vi "PIV_Stats_Single.vi"(0 "Data Folder":path=path "T:/Ensight_Data/NACA0015/NACA0015_NM_B/Test_A", 1 "PIV Meas Plane":enum16{"XY", "YZ", "XZ"}(ring)=enum."XZ", 2 "Row number":i32=1, 5 "Output Directory":path=path "T:/Ensight_Data/NACA0015/NACA0015_NM_B", 7 "XYZ Translation":dbl[](array[numeric])=[200.0, 8.0, -30.0], 9 "Case Name":string="Test_A_Case", 11 "PIV Freq (Hz)":dbl=7.25, 12 "Invert U":bool=TRUE, 13 "Invert V":bool) -> (4 "Progress Bar":i32(slide) scale=0.0..100.0, 6 "Status":string, 10 "# total vectors":i32=9858)   [LabVIEW 2011]
uses:
  <vilib>/Utility/error.llb/DialogType.ctl
  <vilib>/Analysis/1siggen.llb/Ramp Pattern by Samples.vi
  <vilib>/Analysis/NI_AALBase.lvlib
panel:
  out "Max Record Length":i32=3
  out "Tmax":dbl=0.41379310344827586
  out "# vectors without records":i16
  out "Data Array (spot,Var)":dbl[][](array[numeric])
  out "File Paths":path[](array[path])
  out "Position Array (XYZ,spot)":dbl[][](array[numeric])
  out "Variable Names":string[](array[string])=["Record_Length", "CHC", "u_ms", "v_ms", "time_s", "Vel_mag_ms", "Turb_Stats_U_ms", "Turb_Stats_u2_m2s2", "Turb_Stats_u3_m3s3", "Turb_Stats_u4_m4s4", "Turb_Stats_TurbU_%", "Turb_Stats_Skew_u", "Turb_Stats_Kurt_u", "Turb_Stats_V_ms", "Turb_Stats_v2_m2s2", "Turb_Stats_v3_m3s3", "Turb_Stats_v4_m4s4", "Turb_Stats_TurbV_%", "Turb_Stats_Skew_v", "Turb_Stats_Kurt_v", "Turb_Stats_u2v2_m4s4", "Turb_Stats_uv3_m4s4", "Turb_Stats_u3v_m4s4", "Turb_Stats_uv2_m3s3", "Turb_Stats_u2v_m3s3", "Turb_Stats_uv_cc", "Turb_Stats_uv", "Turb_Stats_TKE_J", "Turb_Stats_Error_U_ms", "Turb_Stats_Error_u2_m2s2", "Turb_Stats_Error_u3_m3s3", "Turb_Stats_Error_u4_m4s4", "Turb_Stats_Error_TurbU_%", "Turb_Stats_Error_Skew_u", "Turb_Stats_Error_Kurt_u", "Turb_Stats_Error_V_ms", "Turb_Stats_Error_v2_m2s2", "Turb_Stats_Error_v3_m3s3", "Turb_Stats_Error_v4_m4s4", "Turb_Stats_Error_TurbV_%", "Turb_Stats_Error_Skew_v", "Turb_Stats_Error_Kurt_v", "Turb_Stats_Error_u2v2_m4s4", "Turb_Stats_Error_uv3_m4s4", "Turb_Stats_Error_u3v_m4s4", "Turb_Stats_Error_uv2_m3s3", "Turb_Stats_Error_u2v_m3s3", "Turb_Stats_Error_uv_cc", "Turb_Stats_Error_uv", "Turb_Stats_Error_TKE_J"]
  out "time s":dbl[](array[numeric])=[0.0, 0.20689655172413793, 0.41379310344827586]
  out "File Array":path[](array[path])=[path "T:/Ensight_Data/NACA0015/NACA0015_NM_A/Test_A_Trans/New folder/Test_A000000.T076.D000.P000.H000.L.vec", path "T:/Ensight_Data/NACA0015/NACA0015_NM_A/Test_A_Trans/New folder/Test_A000001.T076.D000.P000.H000.L.vec", path "T:/Ensight_Data/NACA0015/NACA0015_NM_A/Test_A_Trans/New folder/Test_A000002.T076.D000.P000.H000.L.vec"]
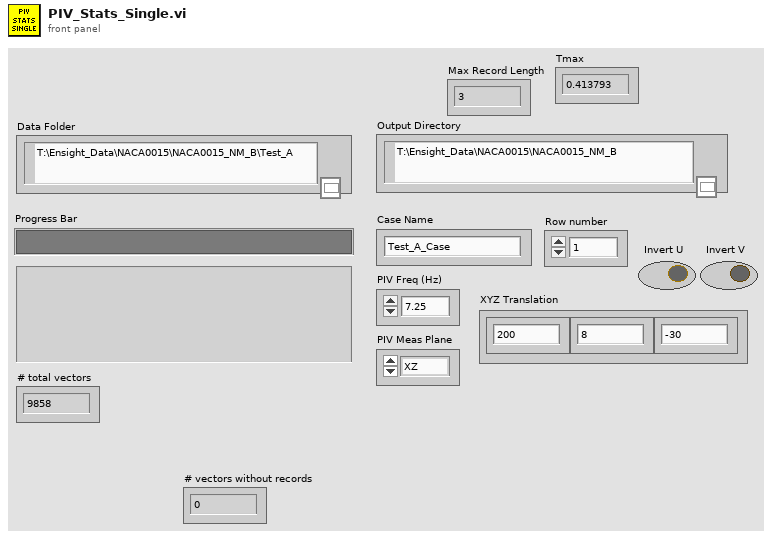
[diagram p1: front panel]
types:
  T1 = cluster{"Record Length":dbl, "CHC":dbl[], "u m/s":dbl[], "v m/s":dbl[], "time s":dbl[], "Vel mag m/s":dbl[], "XYZ Position":dbl[], " Turb Stats":cluster{"U m/s":dbl, "u2 m2/s2":dbl, "u3 m3/s3":dbl, "u4 m4/s4":dbl, "TurbU %":dbl, "Skew_u":dbl, "Kurt_u":dbl, "V m/s":dbl, "v2 m2/s2":dbl, "v3 m3/s3":dbl, "v4 m4/s4":dbl, "TurbV %":dbl, "Skew_v":dbl, "Kurt_v":dbl, "u2v2 m4/s4":dbl, "uv3 m4/s4":dbl, "u3v m4/s4":dbl, "uv2 m3/s3":dbl, "u2v m3/s3":dbl, "uv_cc":dbl, "uv":dbl, "TKE J":dbl}[], "Turb Stats Error":cluster{"U m/s":dbl, "u2 m2/s2":dbl, "u3 m3/s3":dbl, "u4 m4/s4":dbl, "TurbU %":dbl, "Skew_u":dbl, "Kurt_u":dbl, "V m/s":dbl, "v2 m2/s2":dbl, "v3 m3/s3":dbl, "v4 m4/s4":dbl, "TurbV %":dbl, "Skew_v":dbl, "Kurt_v":dbl, "u2v2 m4/s4":dbl, "uv3 m4/s4":dbl, "u3v m4/s4":dbl, "uv2 m3/s3":dbl, "u2v m3/s3":dbl, "uv_cc":dbl, "uv":dbl, "TKE J":dbl}[], "u (good)":dbl[], "v (good)":dbl[]}
  T2 = cluster{"Record Length":dbl, "CHC":dbl[], "u m/s":dbl[], "v m/s":dbl[], "time s":dbl[], "Vel mag m/s":dbl[], "XYZ Position":dbl[], " Turb Stats":cluster{"U m/s":dbl, "u2 m2/s2":dbl, "u3 m3/s3":dbl, "u4 m4/s4":dbl, "TurbU %":dbl, "Skew_u":dbl, "Kurt_u":dbl, "V m/s":dbl, "v2 m2/s2":dbl, "v3 m3/s3":dbl, "v4 m4/s4":dbl, "TurbV %":dbl, "Skew_v":dbl, "Kurt_v":dbl, "u2v2 m4/s4":dbl, "uv3 m4/s4":dbl, "u3v m4/s4":dbl, "uv2 m3/s3":dbl, "u2v m3/s3":dbl, "uv_cc":dbl, "uv":dbl, "TKE J":dbl}[], "Turb Stats Error":cluster{"U m/s":dbl, "u2 m2/s2":dbl, "u3 m3/s3":dbl, "u4 m4/s4":dbl, "TurbU %":dbl, "Skew_u":dbl, "Kurt_u":dbl, "V m/s":dbl, "v2 m2/s2":dbl, "v3 m3/s3":dbl, "v4 m4/s4":dbl, "TurbV %":dbl, "Skew_v":dbl, "Kurt_v":dbl, "u2v2 m4/s4":dbl, "uv3 m4/s4":dbl, "u3v m4/s4":dbl, "uv2 m3/s3":dbl, "u2v m3/s3":dbl, "uv_cc":dbl, "uv":dbl, "TKE J":dbl}[], "u (good)":dbl[], "v (good)":dbl[]}[]
  T3 = cluster{"U m/s":dbl, "u2 m2/s2":dbl, "u3 m3/s3":dbl, "u4 m4/s4":dbl, "TurbU %":dbl, "Skew_u":dbl, "Kurt_u":dbl, "V m/s":dbl, "v2 m2/s2":dbl, "v3 m3/s3":dbl, "v4 m4/s4":dbl, "TurbV %":dbl, "Skew_v":dbl, "Kurt_v":dbl, "u2v2 m4/s4":dbl, "uv3 m4/s4":dbl, "u3v m4/s4":dbl, "uv2 m3/s3":dbl, "u2v m3/s3":dbl, "uv_cc":dbl, "uv":dbl, "TKE J":dbl}
  T4 = cluster{"U m/s":dbl, "u2 m2/s2":dbl, "u3 m3/s3":dbl, "u4 m4/s4":dbl, "TurbU %":dbl, "Skew_u":dbl, "Kurt_u":dbl, "V m/s":dbl, "v2 m2/s2":dbl, "v3 m3/s3":dbl, "v4 m4/s4":dbl, "TurbV %":dbl, "Skew_v":dbl, "Kurt_v":dbl, "u2v2 m4/s4":dbl, "uv3 m4/s4":dbl, "u3v m4/s4":dbl, "uv2 m3/s3":dbl, "u2v m3/s3":dbl, "uv_cc":dbl, "uv":dbl, "TKE J":dbl}[]
  T5 = typedef "DialogType.ctl" = u16
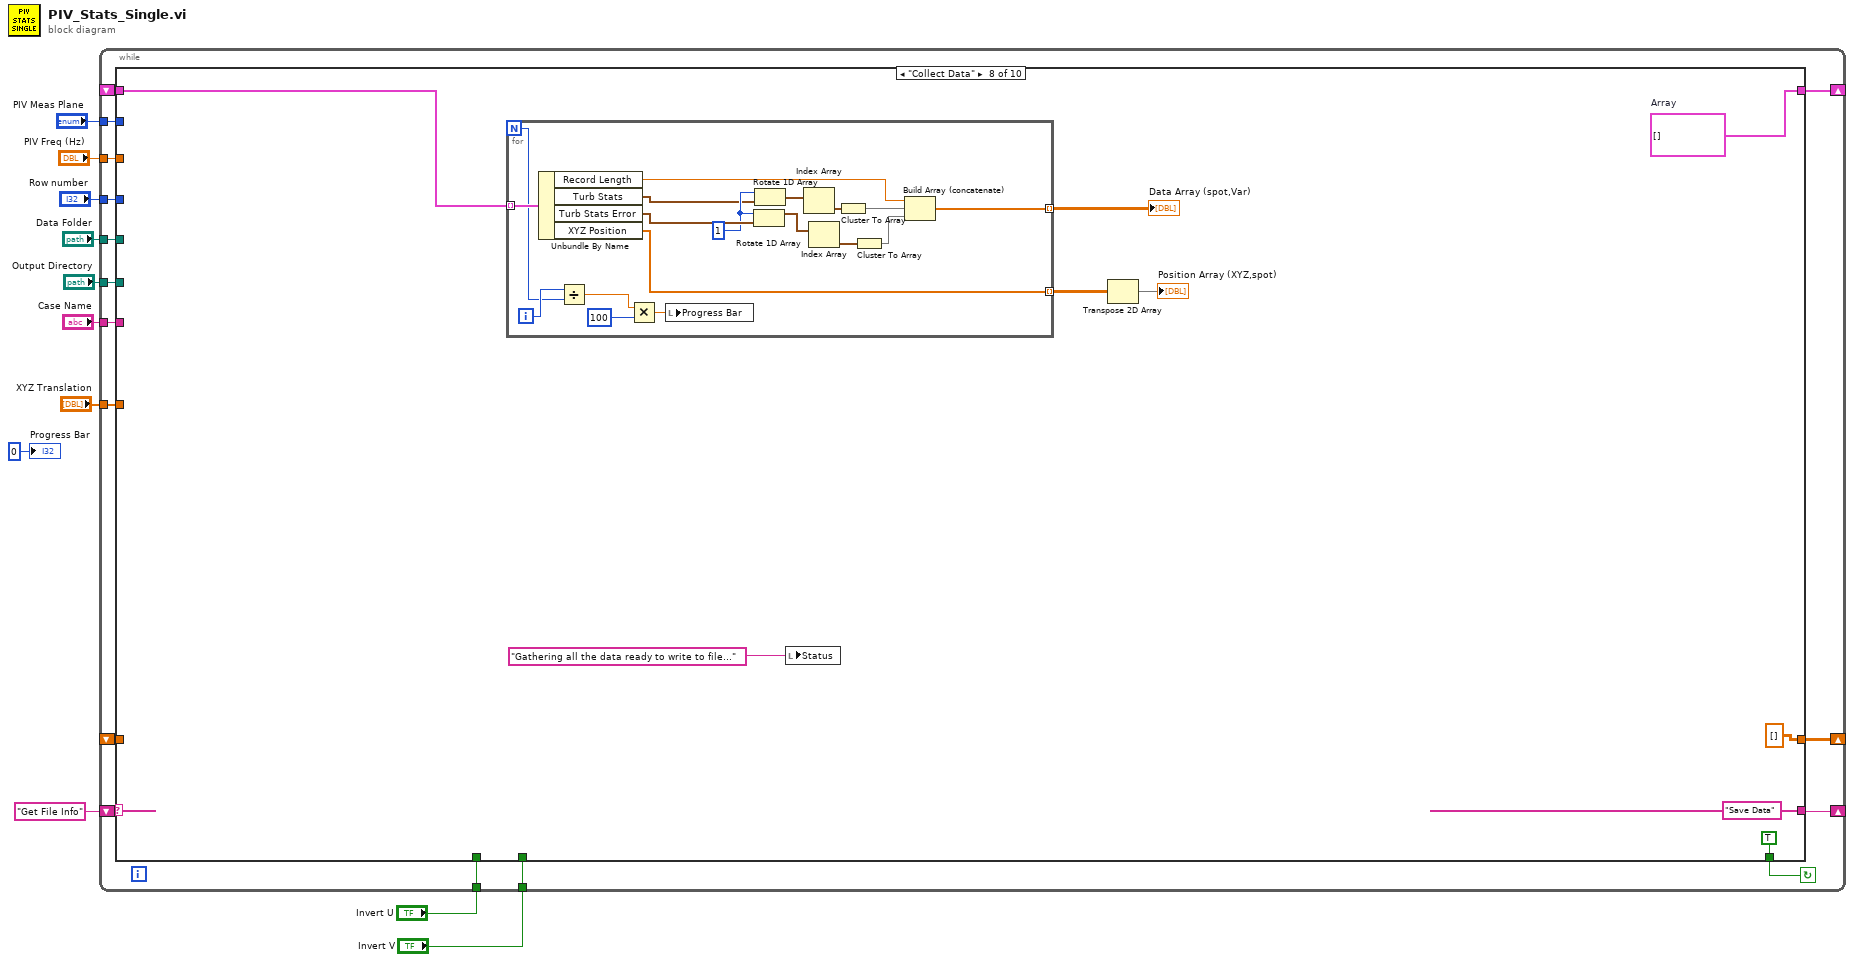
[diagram p0: block diagram]
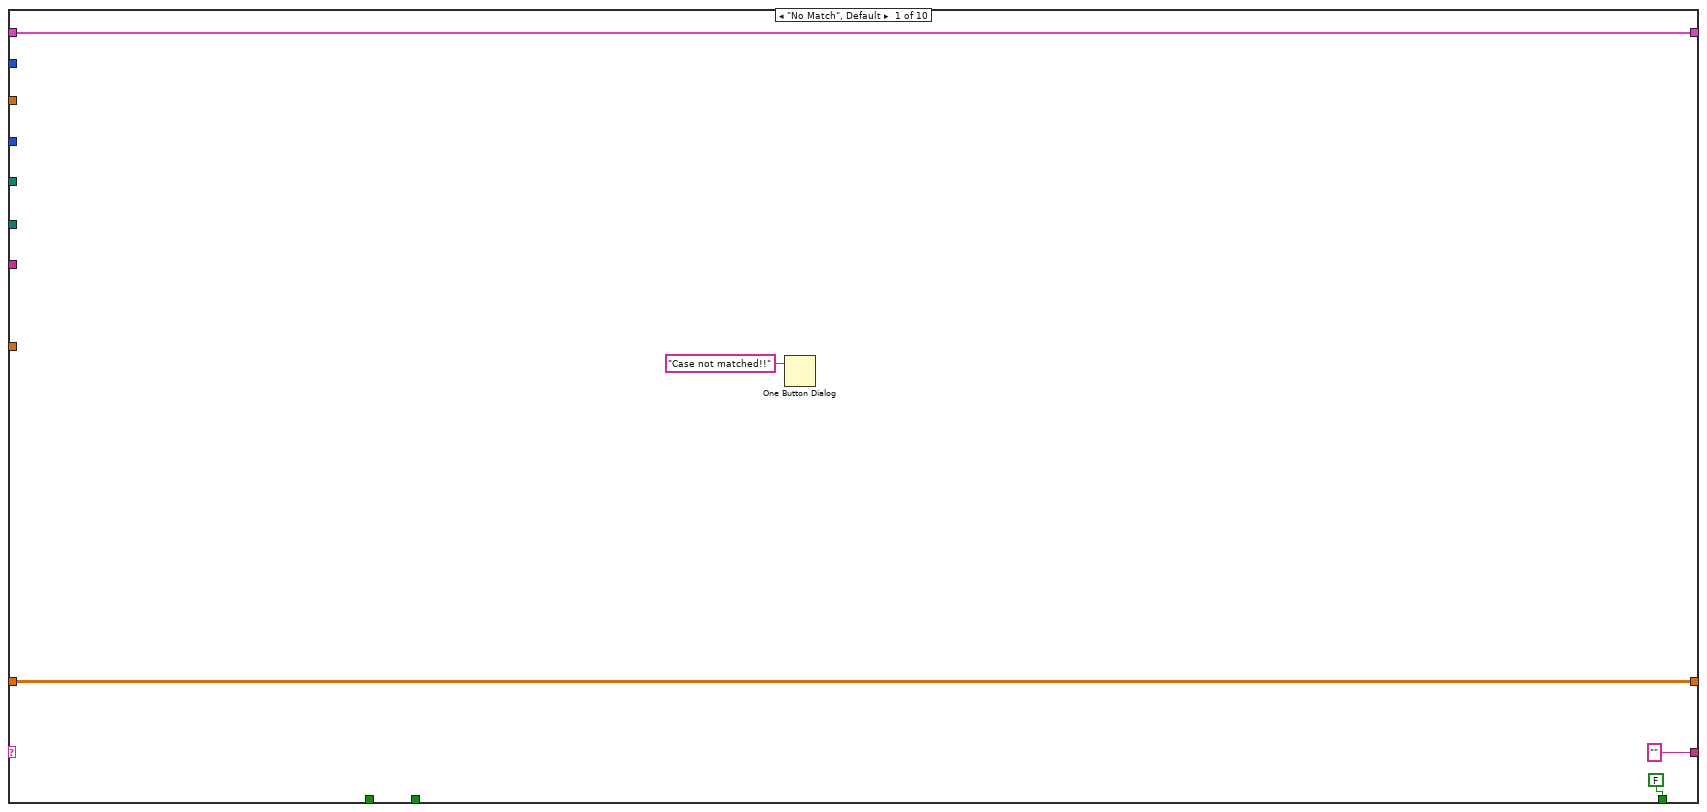
[diagram p2: hidden frame]
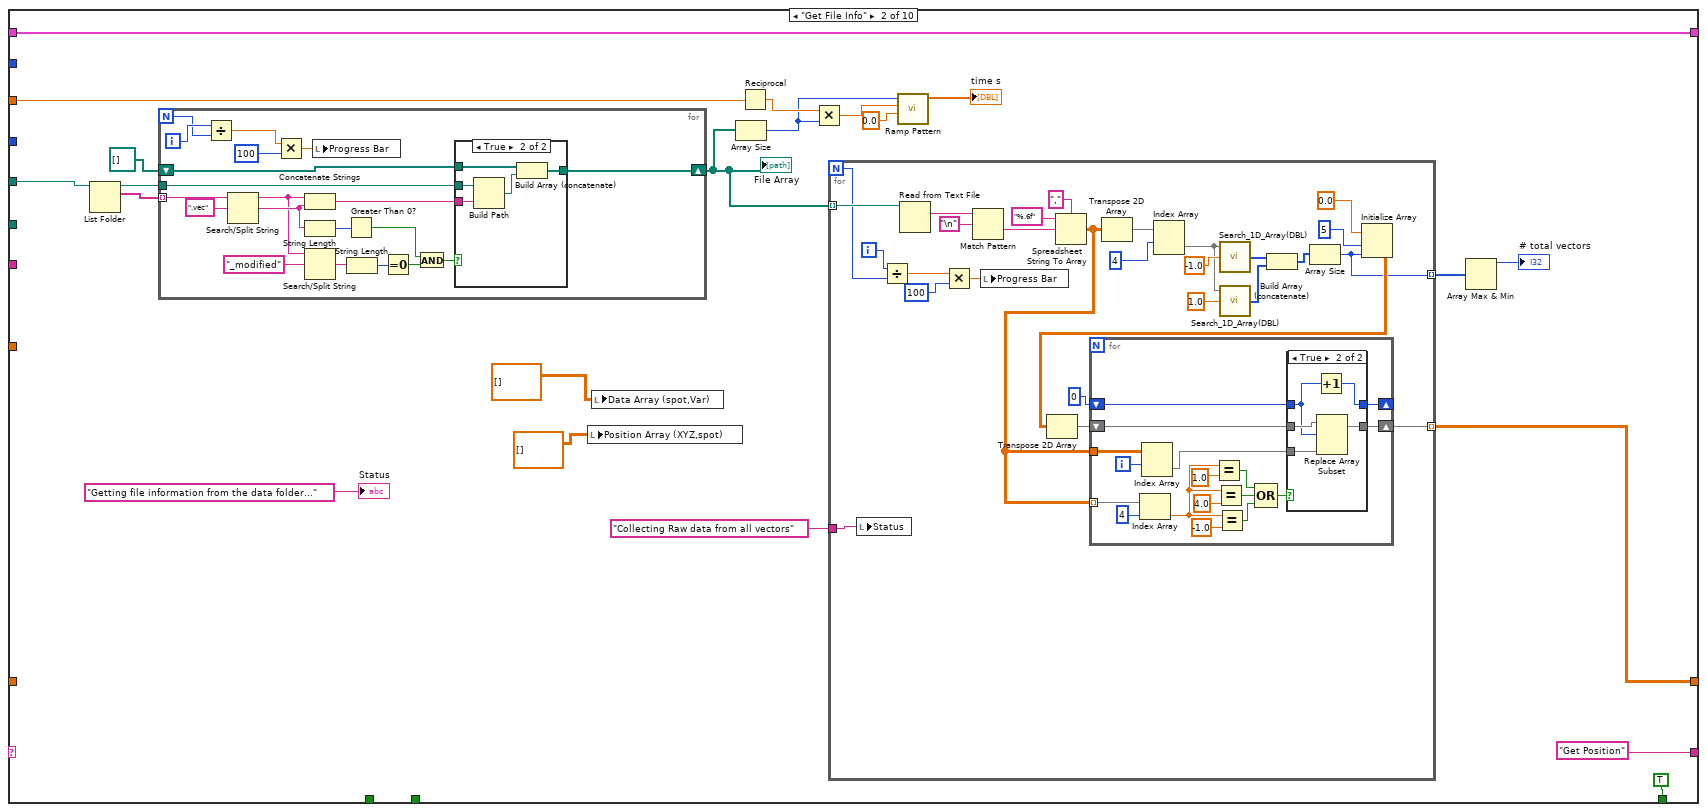
[diagram p3: hidden frame]
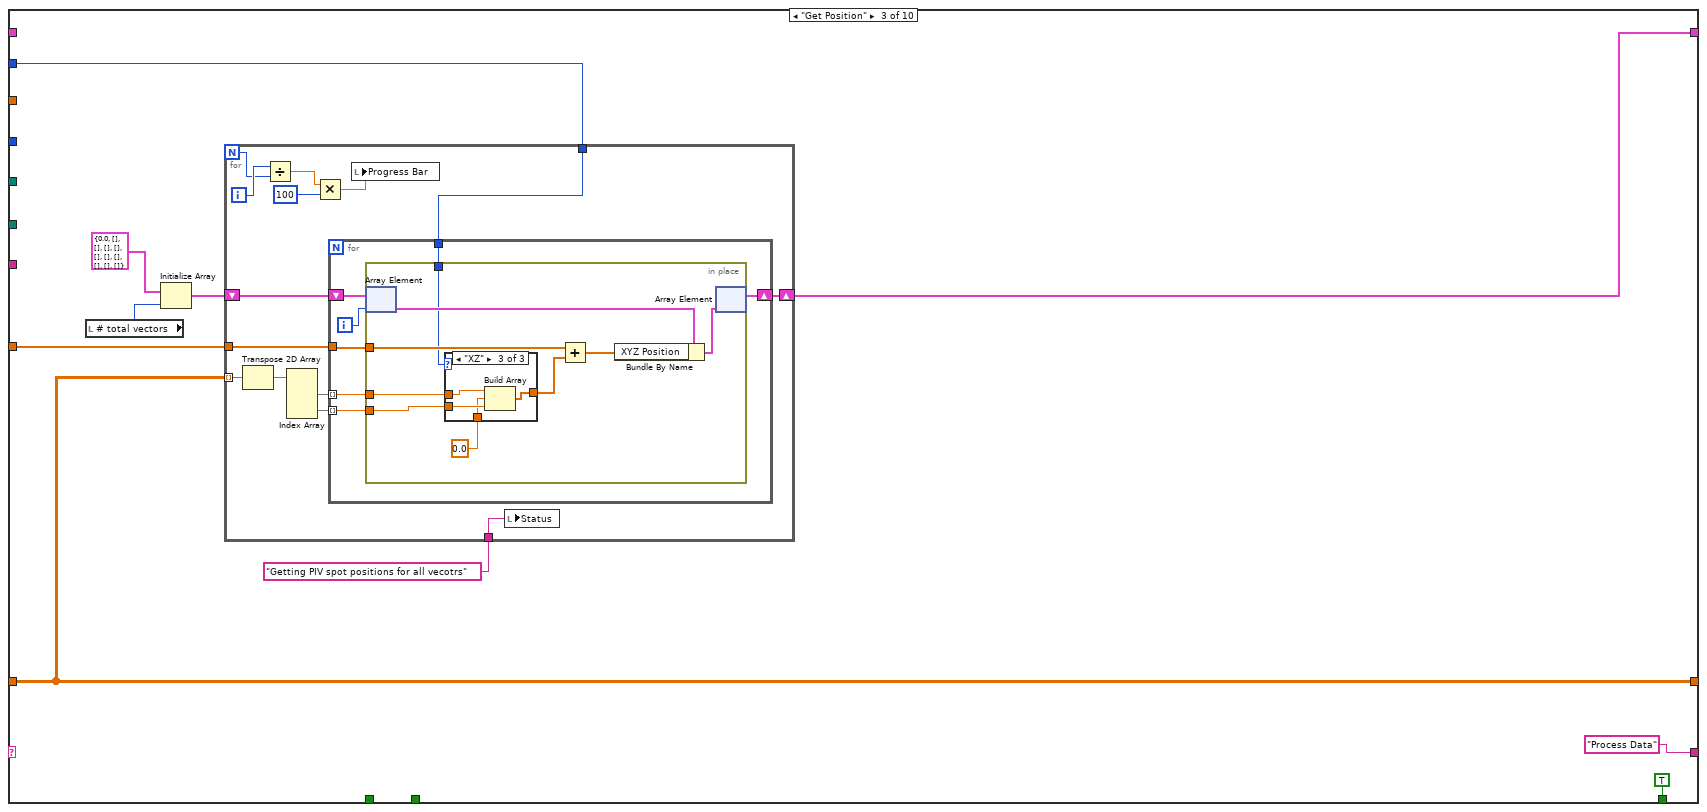
[diagram p6: hidden frame]
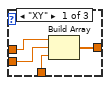
[diagram p7: hidden frame]
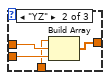
[diagram p8: hidden frame]
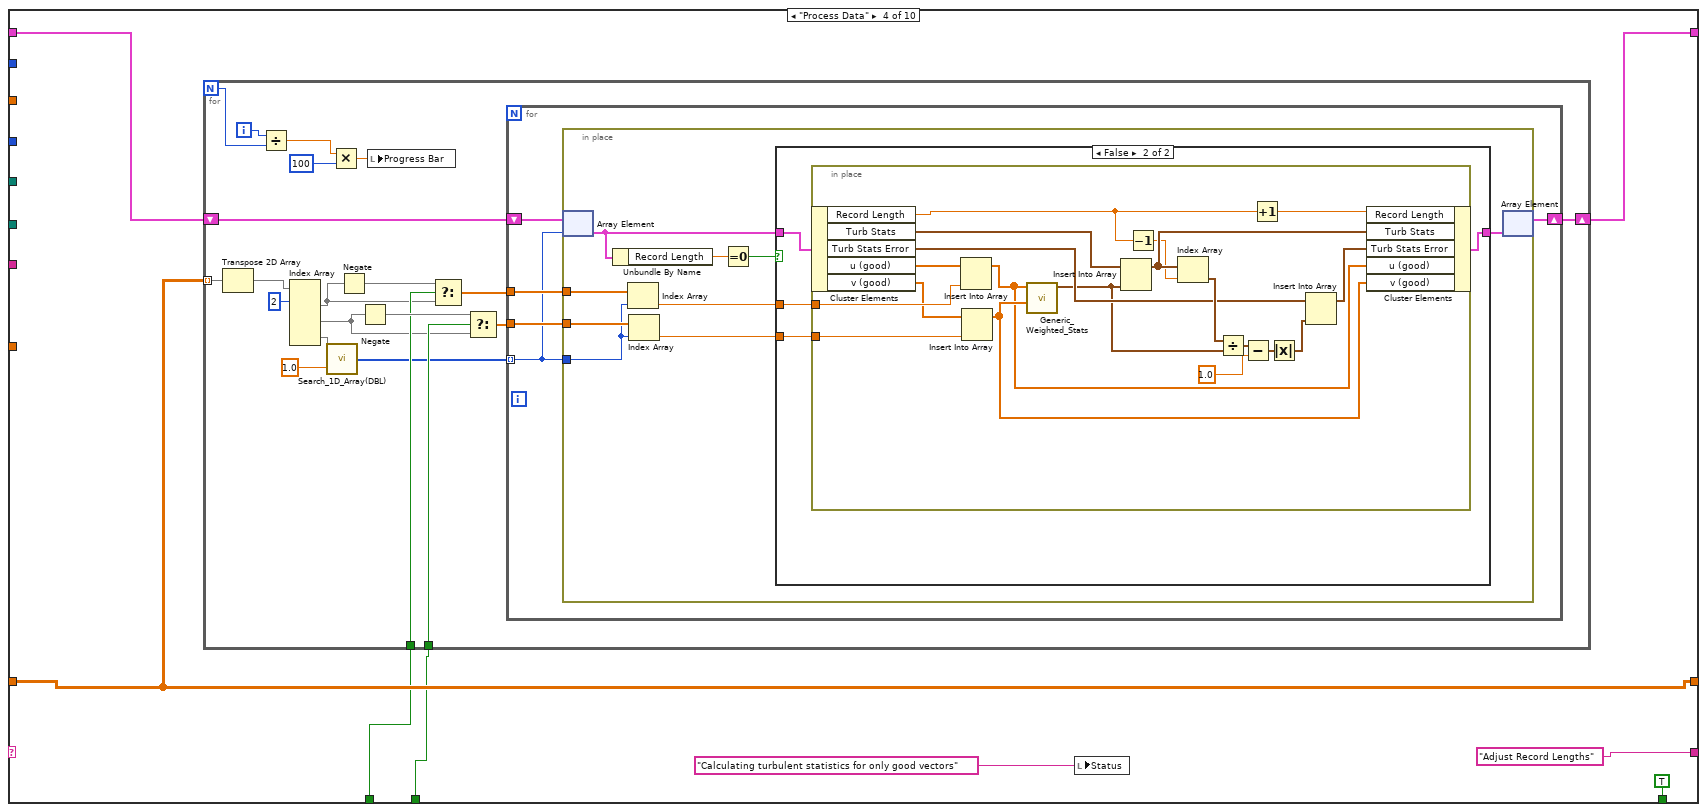
[diagram p9: hidden frame]
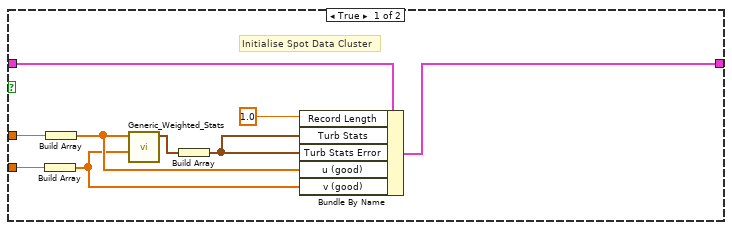
[diagram p10: hidden frame]
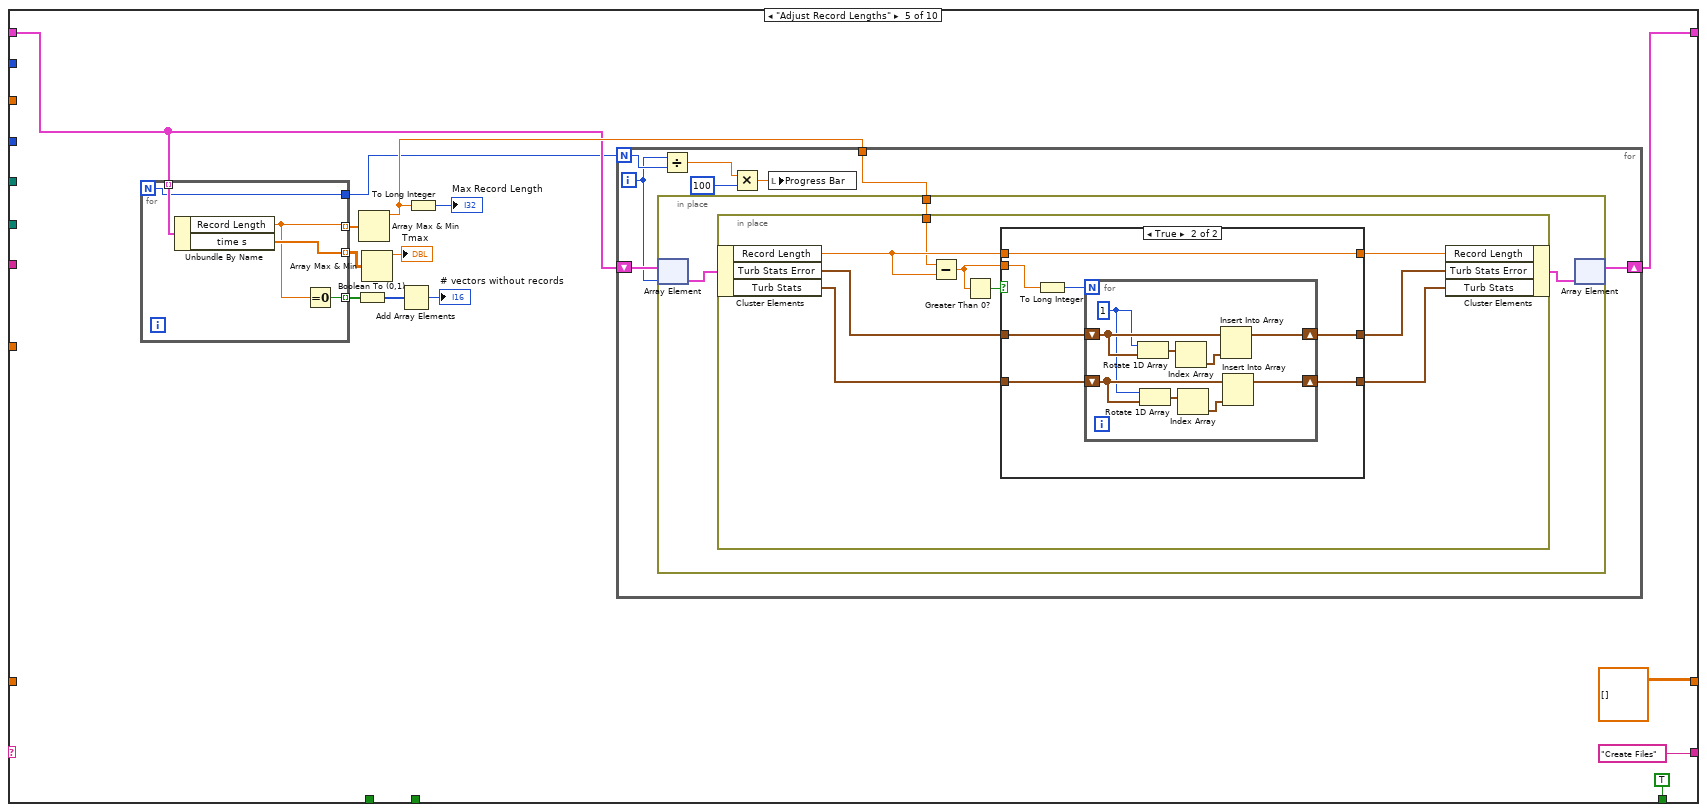
[diagram p11: hidden frame]
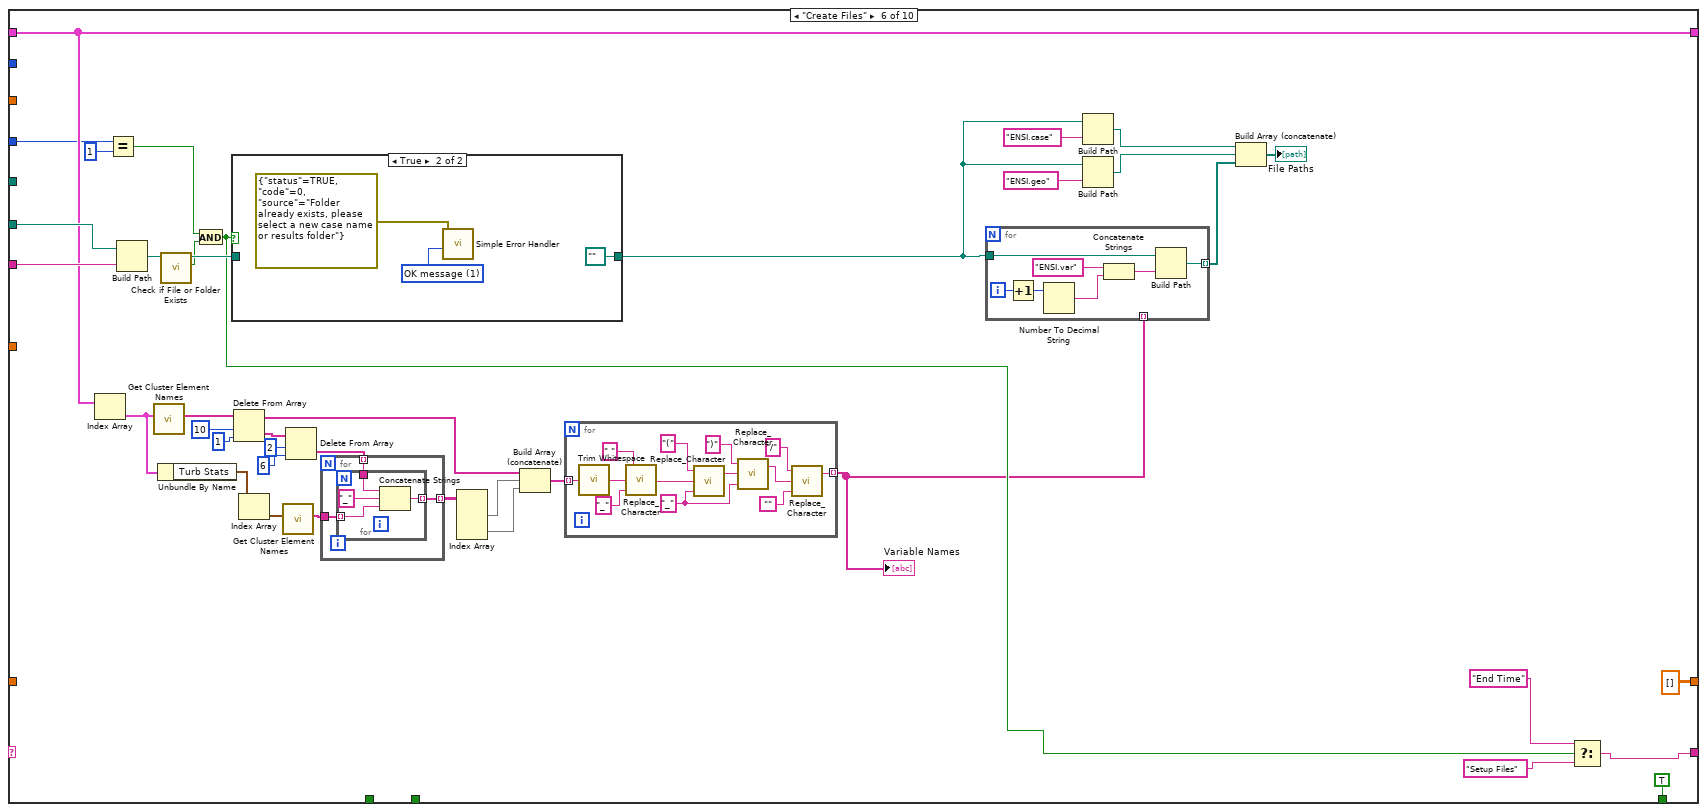
[diagram p13: hidden frame]
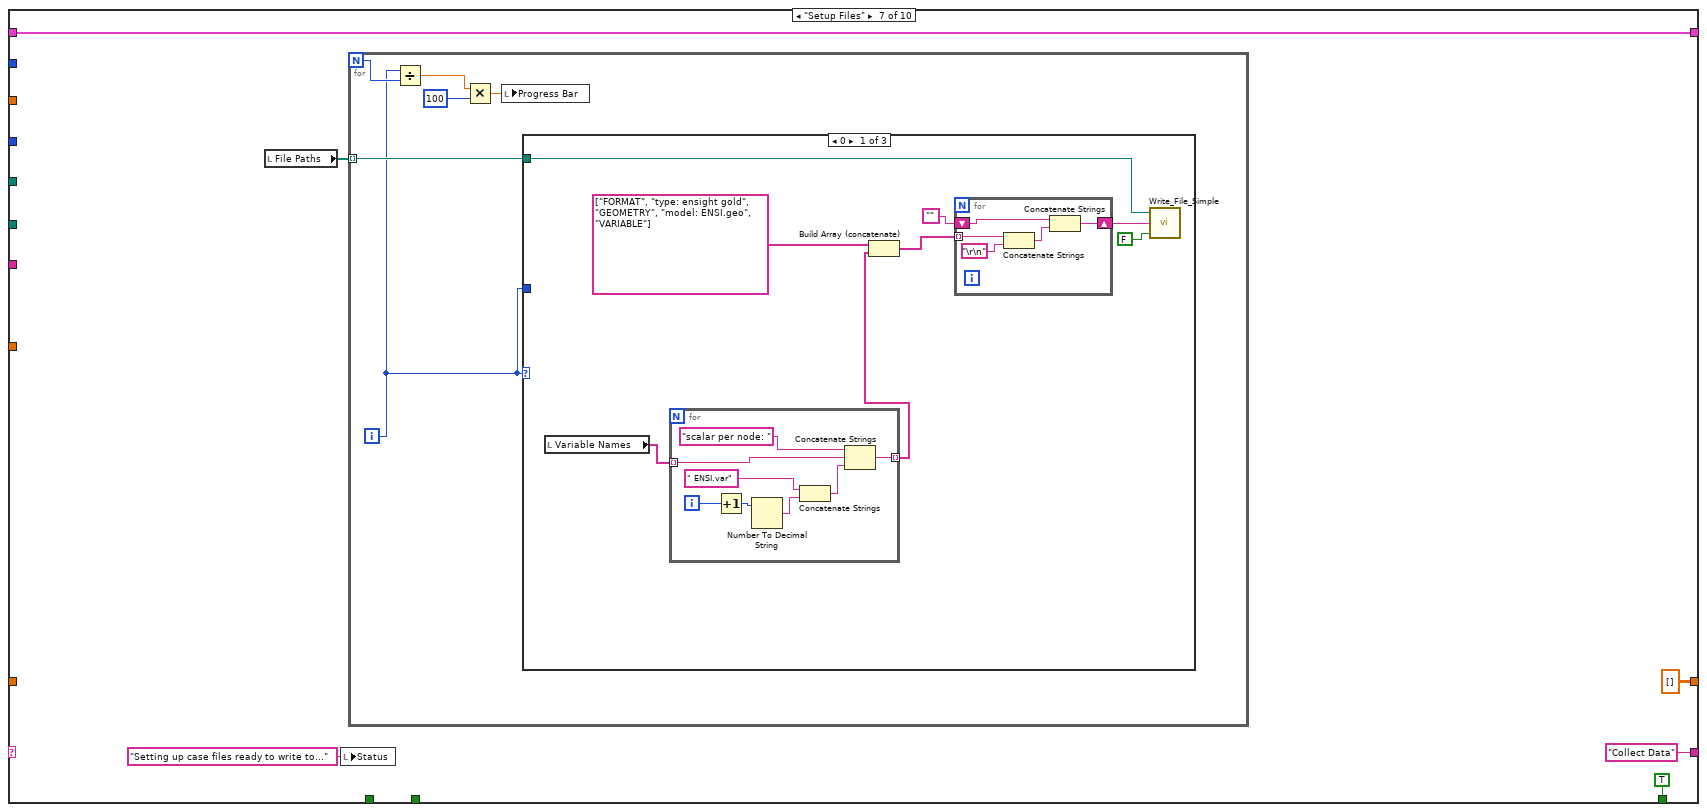
[diagram p15: hidden frame]
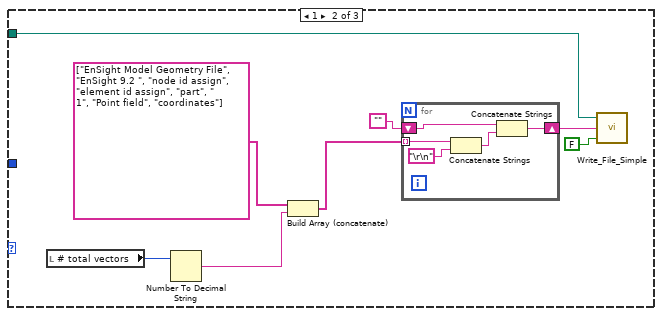
[diagram p16: hidden frame]
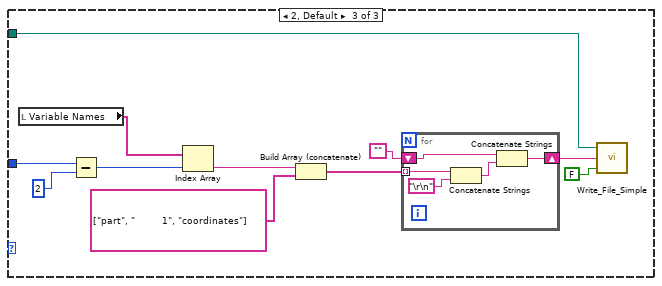
[diagram p17: hidden frame]
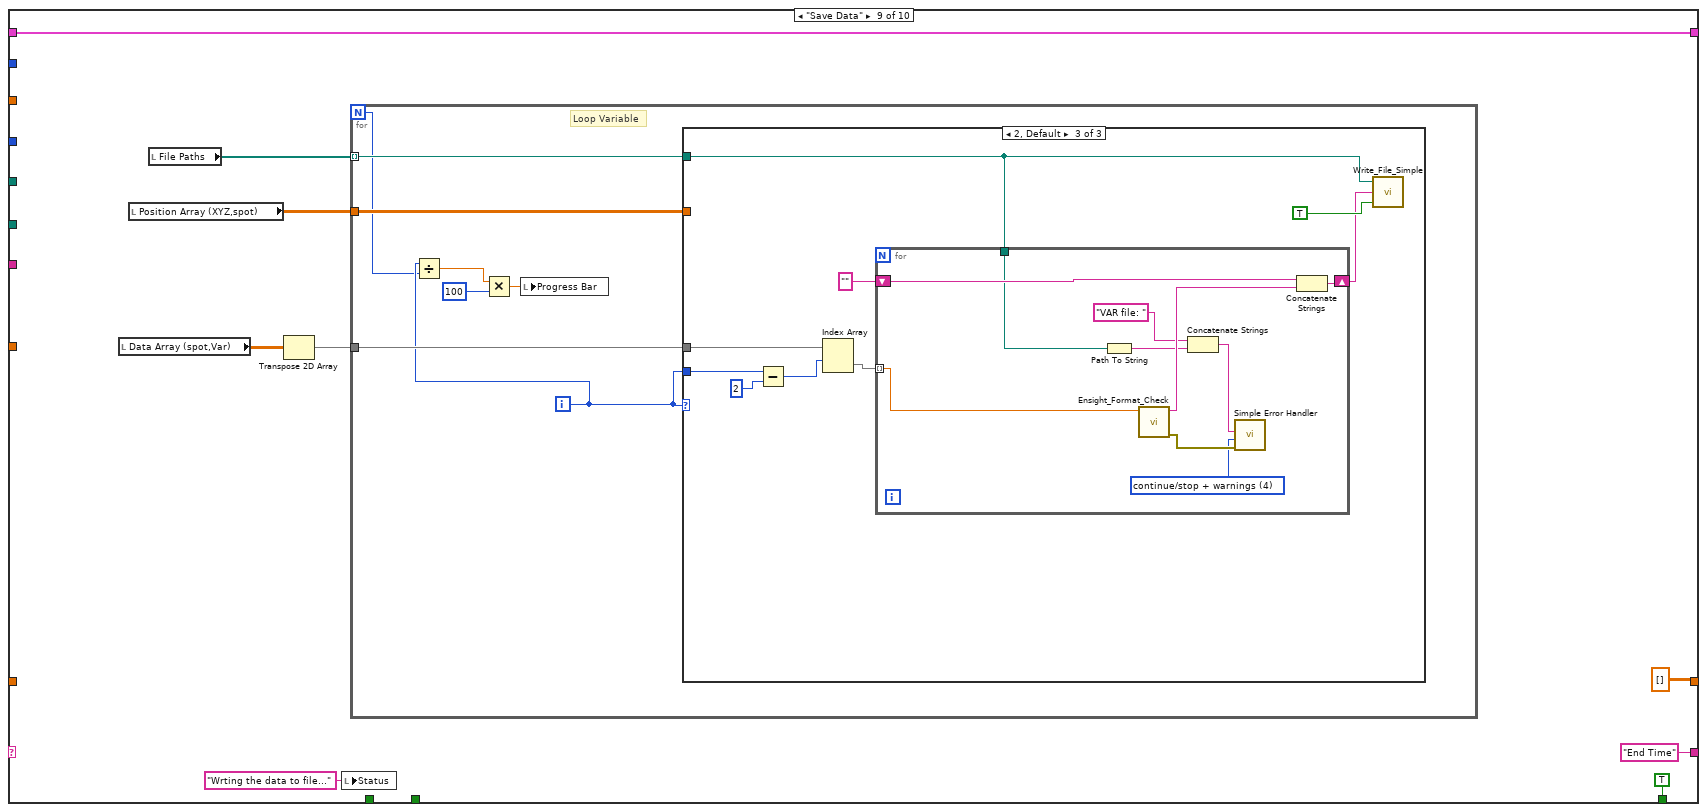
[diagram p18: hidden frame]
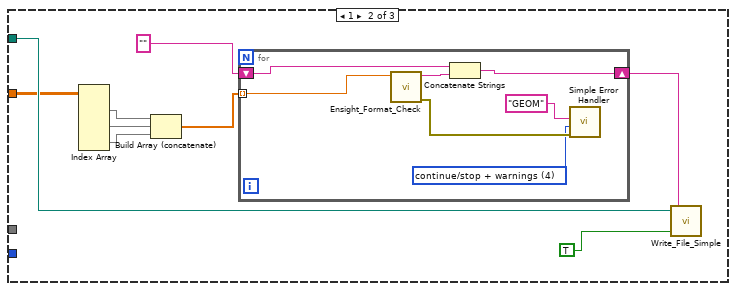
[diagram p20: hidden frame]
diagram:
  n1 = while {
    shift-right: [w26] -> _
    shift-left: "Get File Info" -> [w27]
    tunnel: "Data Folder" -> [w25]
    tunnel: "Output Directory" -> [w23]
    tunnel: "Case Name" -> [w22]
    tunnel: "PIV Freq (Hz)" -> [w21]
    tunnel: "PIV Meas Plane" -> [w20]
    tunnel: "XYZ Translation" -> [w19]
    shift-right: [w18] -> _
    shift-left: _ -> [w17]
    tunnel: "Row number" -> [w16]
    tunnel: "Invert V" -> [w15]
    tunnel: "Invert U" -> [w14]
    shift-right: [w13] -> _
    shift-left: _ -> [w12]
    stop <- w24 continue-if-true
    n2 = case shown="\"Collect Data\"" w27 {
      tunnel: ["" "Get Position" "Process Data" "Adjust Record Lengths" "Create Files" w330 "Collect Data" ("t") "Save Data" ("t") "End Time" ("t") "" ("t")] -> w26
      tunnel: w25 -> [_ w48 _ _ _ _ _ _ _ _]
      tunnel: [FALSE TRUE TRUE TRUE TRUE TRUE TRUE TRUE TRUE FALSE] -> w24
      tunnel: w23 -> [_ _ _ _ _ w354 _ _ _ _]
      tunnel: w22 -> [_ _ _ _ _ w355 _ _ _ _]
      tunnel: w21 -> [_ w47 _ _ _ _ _ _ _ _]
      tunnel: w20 -> [_ _ w138 _ _ _ _ _ _ _]
      tunnel: w19 -> [_ _ w139 _ _ _ _ _ _ _]
      tunnel: [w30 w35 w133 w184 w260 w340 w389 w453 w482 w529] -> w18
      tunnel: w17 -> [w30 w35 _ w188 w262 w340 w389 w455 w482 w529]
      tunnel: w16 -> [_ _ _ _ _ w336 _ _ _ _]
      tunnel: w15 -> [_ _ _ w185 _ _ _ _ _ _]
      tunnel: w14 -> [_ _ _ w186 _ _ _ _ _ _]
      tunnel: [w28 w33 w132 w187 dbl[][][] [] ("GoodRawData(time,spot)") dbl[][][] [] ("GoodRawData(time,spot)") dbl[][][] [] ("GoodRawData(time,spot)") dbl[][][] [] ("GoodRawData(time,spot)") dbl[][][] [] ("GoodRawData(time,spot)") w528] -> w13
      tunnel: w12 -> [w28 _ w132 w187 _ _ _ _ _ w528]
      frame "No Match", Default {
        n3 = One Button Dialog(message="Case not matched!!") -> ()  [unwired: 1 in, 1 out]
      }
      frame "Get File Info" {
        n4 = List Folder(path=w48) -> (path out=w50:path, filenames=w51:string[])  [unwired: 3 in, 2 out]
        n5 = for {
          N -> [w106]
          tunnel: w51 -> [w125] mode=indexing
          shift-right: [w118] -> w38
          shift-left: path[] [] -> [w120]
          tunnel: w50 -> [w119]
          i -> [w107]
          n6 = Divide(x=w107, y=w106) -> (x/y=w109:dbl)
          n7 = Search/Split String(string=w125, search string/char (-)=".vec") -> (substring before match=w116:string, match + rest of string=w122:string)  [unwired: 1 in, 1 out]
          n8 = Multiply(x=w109, y=100) -> (x*y=w110:dbl)
          n9 = Concatenate Strings(w116, w122) -> (w121:string)
          n10 = String Length(string=w122) -> (length=w123:i32)
          n11 = Search/Split String(string=w116, search string/char (-)="_modified") -> (match + rest of string=w114:string)  [unwired: 1 in, 2 out]
          n12 = local write "Progress Bar"(w110) -> ()
          n13 = Greater Than 0?(x=w123) -> (x > 0?=w117:bool)
          n14 = String Length(string=w114) -> (length=w113:i32)
          n15 = Equal To 0?(x=w113) -> (x = 0?=w112:bool)
          n16 = And(x=w117, y=w112) -> (x .and. y?=w111:bool)
          n17 = case shown="True" w111 {
            tunnel: w121 -> [_ w131]
            tunnel: w120 -> [w126 w127]
            tunnel: w119 -> [_ w130]
            tunnel: [w126 w128] -> w118
            frame False {
            }
            frame True {
              n18 = Build Path(base path=w130, name or relative path=w131) -> (appended path=w129:path)
              n19 = Build Array (concatenate)(w127, w129) -> (w128:path[])
            }
          }
        }
        "File Array" <- w38
        n20 = local write "Position Array (XYZ,spot)"(dbl[][] [] ("Position Array")) -> ()
        n21 = local write "Data Array (spot,Var)"(dbl[][] [] ("Data Array")) -> ()
        n22 = Array Size(array=w38) -> (size(s)=w42:i32)
        n23 = Reciprocal(x=w47) -> (1/x=w45:dbl)
        n24 = Multiply(x=w45, y=w42) -> (x*y=w46:dbl)
        n25 = for {
          N -> [w65]
          tunnel: w38 -> [w72] mode=indexing
          tunnel: [w54] -> w37 mode=indexing
          tunnel: [w69] -> w33 mode=indexing
          tunnel: "Collecting Raw data from all vectors" ("Status") -> [w63]
          i -> [w64]
          n26 = local write "Status"(w63) -> ()
          n27 = Divide(x=w64, y=w65) -> (x/y=w67:dbl)
          n28 = Read from Text File(file (use dialog)=w72) -> (text=w81:string)  [unwired: 3 in, 3 out]
          n29 = Multiply(x=w67, y=100) -> (x*y=w66:dbl)
          n30 = Match Pattern(string=w81, regular expression="\n") -> (after substring=w77:string)  [unwired: 1 in, 3 out]
          n31 = local write "Progress Bar"(w66) -> ()
          n32 = Spreadsheet String To Array(delimiter (Tab)=",", format string="%.6f", spreadsheet string=w77) -> (array=w60:dbl[][])  [unwired: 1 in]
          n33 = Transpose 2D Array(2D array=w60) -> (transposed array=w76:dbl[][])
          n34 = Index Array(array=w76, index (row)=4) -> (element=w59:dbl[])  [unwired: 1 in]
          n35 = call "Search_1D_Array(DBL).vi"("Array"=w59, "Element Data"=-1.0) -> ("Indicies of Elements"=w58:i32[])  [unwired: 7 in]
          n36 = call "Search_1D_Array(DBL).vi"("Array"=w59, "Element Data"=1.0) -> ("Indicies of Elements"=w56:i32[])  [unwired: 7 in]
          n37 = Build Array (concatenate)(w58, w56) -> (w57:i32[])
          n38 = Array Size(array=w57) -> (size(s)=w54:i32)
          n39 = Initialize Array(0.0 ("element"), 5 ("dimension size"), w54) -> (w70:dbl[][])
          n40 = Transpose 2D Array(2D array=w70) -> (transposed array=w71:dbl[][])
          n41 = for {
            tunnel: w60 -> [w93] mode=indexing
            shift-right: [w96] -> w69
            shift-left: w71 -> [w91]
            shift-right: [w95] -> _
            shift-left: 0 ("y") -> [w94]
            tunnel: w60 -> [w92]
            i -> [w90]
            n42 = Index Array(array=w93, index=4) -> (element=w87:dbl)
            n43 = Index Array(array=w92, index (row)=w90) -> (element=w97:dbl[])  [unwired: 1 in]
            n44 = Equal?(x=w87, y=1.0) -> (x = y?=w83:bool)
            n45 = Equal?(x=w87, y=4.0) -> (x = y?=w84:bool)
            n46 = Equal?(x=w87, y=-1.0) -> (x = y?=w85:bool)
            n47 = Compound Arithmetic op=OR(w83, w84, w85) -> (w82:bool)
            n48 = case shown="True" w82 {
              tunnel: w97 -> [_ w103]
              tunnel: w91 -> [w100 w105]
              tunnel: [w100 w104] -> w96
              tunnel: [w99 w102] -> w95
              tunnel: w94 -> [w99 w101]
              frame False {
              }
              frame True {
                n49 = Increment(x=w101) -> (x+1=w102:i32)
                n50 = Replace Array Subset(array=w105, new element=w103, index (row)=w101) -> (w104:dbl[][])  [unwired: 1 in]
              }
            }
          }
        }
        n51 = call-poly <vilib>:"Ramp Pattern.vi"("start"=0.0, "end"=w46, "samples"=w42) -> ("Ramp Pattern"=→"time s":dbl[])  [unwired: 7 in, 1 out]
        n52 = Array Max & Min(array=w37) -> (max value=→"# total vectors":i32)  [unwired: 3 out]
        "Status" <- "Getting file information from the data folder..." ("Status")
      }
      frame "Get Position" {
        n53 = local read "# total vectors"() -> (w137:i32)
        n54 = Initialize Array(T1 {"Record Length"=0.0, "CHC"=[], "u m/s"=[], "v m/s"=[], "time s"=[], "Vel mag m/s"=[], "XYZ Position"=[], " Turb Stats"=[], "Turb Stats Error"=[], "u (good)"=[], "v (good)"=[]} ("Spot Data Cluster"), w137) -> (w135:T2)
        n55 = for {
          N -> [w146]
          shift-right: [w151] -> w133
          shift-left: w135 -> [w152]
          tunnel: w132 -> [w144] mode=indexing
          tunnel: w139 -> [w153]
          tunnel: w138 -> [w145]
          tunnel: "Getting PIV spot positions for all vecotrs" ("Status") -> [w142]
          i -> [w147]
          n56 = Transpose 2D Array(2D array=w144) -> (transposed array=w143:dbl[][])
          n57 = Divide(x=w147, y=w146) -> (x/y=w149:dbl)
          n58 = Index Array(array=w143) -> (element #1=w155:dbl[], element #2=w154:dbl[])  [unwired: 4 in]
          n59 = Multiply(x=w149, y=100) -> (x*y=w150:dbl)
          n60 = for {
            tunnel: w155 -> [w162] mode=indexing
            tunnel: w154 -> [w161] mode=indexing
            tunnel: w153 -> [w160]
            shift-right: [w157] -> w151
            shift-left: w152 -> [w159]
            tunnel: w145 -> [w156]
            i -> [w158]
            n61 = in-place {
              in-place-border: w162 -> [w169]
              in-place-border: w161 -> [w168]
              in-place-border: w160 -> [w167]
              in-place-border: w156 -> [w163]
              n62 = in-place-array #1(w159, w158) -> (w166:T1)
              n63 = case shown="\"XZ\"" w163 {
                tunnel: w169 -> [w173 w179 w183]
                tunnel: w168 -> [w174 w178 w182]
                tunnel: 0.0 ("element") -> [w175 w177 w181]
                tunnel: [w172 w176 w180] -> w171
                frame "XY" {
                  n64 = Build Array(w173, w174, w175) -> (w172:dbl[])
                }
                frame "YZ" {
                  n65 = Build Array(w177, w179, w178) -> (w176:dbl[])
                }
                frame "XZ" {
                  n66 = Build Array(w183, w181, w182) -> (w180:dbl[])
                }
              }
              n67 = Add(x=w167, y=w171) -> (x+y=w165:dbl[])
              n68 = Bundle By Name(cluster=w166, "XYZ Position"=w165) -> (w164:T1)
              n69 = in-place-array #1(w164) -> (w157:T2)  [unwired: 1 out]
            }
          }
          n70 = local write "Progress Bar"(w150) -> ()
          n71 = local write "Status"(w142) -> ()
        }
      }
      frame "Process Data" {
        n72 = for {
          N -> [w202]
          tunnel: w185 -> [w200]
          tunnel: w186 -> [w199]
          tunnel: w187 -> [w198] mode=indexing
          shift-right: [w207] -> w184
          shift-left: w188 -> [w212]
          i -> [w201]
          n73 = Transpose 2D Array(2D array=w198) -> (transposed array=w197:dbl[][])
          n74 = Divide(x=w201, y=w202) -> (x/y=w204:dbl)
          n75 = Index Array(array=w197, index (row) #1=2 ("index (row)")) -> (element #1=w195:dbl[], element #2=w194:dbl[], element #3=w193:dbl[])  [unwired: 5 in]
          n76 = call "Search_1D_Array(DBL).vi"("Array"=w193, "Element Data"=1.0) -> ("Indicies of Elements"=w192:i32[])  [unwired: 7 in]
          n77 = Multiply(x=w204, y=100) -> (x*y=w205:dbl)
          n78 = Negate(x=w195) -> (-x=w211:dbl[])
          n79 = Negate(x=w194) -> (-x=w210:dbl[])
          n80 = local write "Progress Bar"(w205) -> ()
          n81 = Select(t=w211, s=w199, f=w195) -> (s? t:f=w209:dbl[])
          n82 = Select(t=w210, s=w200, f=w194) -> (s? t:f=w208:dbl[])
          n83 = for {
            tunnel: w209 -> [w217]
            tunnel: w208 -> [w216]
            tunnel: w192 -> [w213] mode=indexing
            shift-right: [w214] -> w207
            shift-left: w212 -> [w215]
            n84 = in-place {
              in-place-border: w217 -> [w226]
              in-place-border: w216 -> [w225]
              in-place-border: w213 -> [w218]
              n85 = in-place-array #2(w215, w213) -> (w220:T1)
              n86 = Unbundle By Name(w220) -> ("Record Length"=w221:dbl)
              n87 = Index Array(array=w226, index=w218) -> (element=w223:dbl)
              n88 = Index Array(array=w225, index=w218) -> (element=w222:dbl)
              n89 = Equal To 0?(x=w221) -> (x = 0?=w224:bool)
              n90 = case shown="False" w224 {
                tunnel: [w234 w239] -> w219
                tunnel: w222 -> [w229 w236]
                tunnel: w220 -> [w235 w238]
                tunnel: w223 -> [w230 w237]
                frame True {
                  # "Initialise Spot Data Cluster"
                  n91 = Build Array(w229) -> (w227:dbl[])
                  n92 = Build Array(w230) -> (w228:dbl[])
                  n93 = call "Generic_Weighted_Stats.vi"("v"=w227, "u"=w228) -> ("Turbulence Statistics"=w232:T3)  [unwired: 9 in]
                  n94 = Build Array(w232) -> (w231:T4)
                  n95 = Bundle By Name(cluster=w235, "Record Length"=1.0, "Turb Stats"=w231, "Turb Stats Error"=w231, "u (good)"=w228, "v (good)"=w227) -> (w234:T1)
                }
                frame False {
                  n96 = in-place {
                    in-place-border: w237 -> [w245]
                    in-place-border: w236 -> [w244]
                    n97 = in-place-cluster #3(w238) -> ("Record Length"=w256:dbl, "Turb Stats"=w258:T4, "Turb Stats Error"=w248:T4, "u (good)"=w246:dbl[], "v (good)"=w243:dbl[])
                    n98 = Insert Into Array(array=w246, new element=w245) -> (w241:dbl[])  [unwired: 1 in]
                    n99 = Insert Into Array(array=w243, new element=w244) -> (w242:dbl[])  [unwired: 1 in]
                    n100 = call "Generic_Weighted_Stats.vi"("v"=w242, "u"=w241) -> ("Turbulence Statistics"=w247:T3)  [unwired: 9 in]
                    n101 = Insert Into Array(array=w258, new element=w247) -> (w257:T4)  [unwired: 1 in]
                    n102 = Decrement(x=w256) -> (x-1=w255:dbl)
                    n103 = Index Array(array=w257, index=w255) -> (element=w254:T3)
                    n104 = Divide(x=w254, y=w247) -> (x/y=w253:T3)
                    n105 = Subtract(x=w253, y=1.0 ("Record Length")) -> (x-y=w251:T3)
                    n106 = Increment(x=w256) -> (x+1=w249:dbl)
                    n107 = Absolute Value(x=w251) -> (abs(x)=w240:T3)
                    n108 = Insert Into Array(array=w248, new element=w240) -> (w250:T4)  [unwired: 1 in]
                    n109 = in-place-cluster #3("Record Length"=w249, "Turb Stats"=w257, "Turb Stats Error"=w250, "u (good)"=w241, "v (good)"=w242) -> (w239:T1)
                  }
                }
              }
              n110 = in-place-array #2(w219) -> (w214:T2)  [unwired: 1 out]
            }
          }
        }
        n111 = local write "Status"("Calculating turbulent statistics for only good vectors" ("Status")) -> ()
      }
      frame "Adjust Record Lengths" {
        n112 = for {
          N -> [w273]
          tunnel: w262 -> [w277] mode=indexing
          tunnel: [w275] -> w263 mode=indexing
          tunnel: [w276] -> w266 mode=indexing
          tunnel: [w274] -> w268 mode=indexing
          tunnel: [w273] -> w259
          n113 = Unbundle By Name(w277) -> ("Record Length"=w275:dbl, "time s"=w276:dbl[])
          n114 = Equal To 0?(x=w275) -> (x = 0?=w274:bool)
        }
        n115 = Boolean To (0,1)(Boolean=w268) -> (0, 1=w269:i16[])
        n116 = Array Max & Min(array=w263) -> (max value=w264:dbl)  [unwired: 3 out]
        n117 = Array Max & Min(array=w266) -> (max value=→"Tmax":dbl)  [unwired: 3 out]
        n118 = Add Array Elements(numeric array=w269) -> (sum=→"# vectors without records":i16)
        n119 = To Long Integer(number=w264) -> (32bit integer=→"Max Record Length":i32)
        n120 = for {
          N: w259 -> [w283]
          tunnel: w264 -> [w285]
          shift-right: [w279] -> w260
          shift-left: w262 -> [w280]
          i -> [w278]
          n121 = in-place {
            in-place-border: w285 -> [w288]
            n122 = in-place-array #4(w280, w278) -> (w287:T1)
            n123 = in-place {
              in-place-border: w288 -> [w289]
              n124 = in-place-cluster #5(w287) -> ("Record Length"=w290:dbl, "Turb Stats Error"=w293:T4, "Turb Stats"=w291:T4)
              n125 = Subtract(x=w289, y=w290) -> (x-y=w296:dbl)
              n126 = Greater Than 0?(x=w296) -> (x > 0?=w297:bool)
              n127 = case shown="True" w297 {
                tunnel: w296 -> [_ w307]
                tunnel: [w298 w301] -> w295
                tunnel: [w300 w304] -> w294
                tunnel: w293 -> [w300 w306]
                tunnel: [w299 w303] -> w292
                tunnel: w291 -> [w299 w305]
                tunnel: w290 -> [w298 w301]
                frame False {
                }
                frame True {
                  n128 = To Long Integer(number=w307) -> (32bit integer=w302:i32)
                  n129 = for {
                    N: w302 -> [_]
                    shift-right: [w313] -> w304
                    shift-left: w306 -> [w314]
                    shift-right: [w312] -> w303
                    shift-left: w305 -> [w311]
                    w308 = 1 ("n")
                    n130 = Rotate 1D Array(1:w314, 2:w308) -> (0:w315:T4)
                    n131 = Rotate 1D Array(1:w311, 2:w308) -> (0:w310:T4)
                    n132 = Index Array(array=w315) -> (element=w316:T3)  [unwired: 1 in]
                    n133 = Index Array(array=w310) -> (element=w309:T3)  [unwired: 1 in]
                    n134 = Insert Into Array(array=w314, new element=w316) -> (w313:T4)  [unwired: 1 in]
                    n135 = Insert Into Array(array=w311, new element=w309) -> (w312:T4)  [unwired: 1 in]
                  }
                }
              }
              n136 = in-place-cluster #5("Record Length"=w295, "Turb Stats Error"=w294, "Turb Stats"=w292) -> (w286:T1)
            }
            n137 = in-place-array #4(w286) -> (w279:T2)  [unwired: 1 out]
          }
          n138 = Divide(x=w278, y=w283) -> (x/y=w282:dbl)
          n139 = Multiply(x=w282, y=100) -> (x*y=w284:dbl)
          n140 = local write "Progress Bar"(w284) -> ()
        }
      }
      frame "Create Files" {
        n141 = Index Array(array=w340) -> (element=w352:T1)  [unwired: 1 in]
        n142 = Equal?(x=w336, y=1) -> (x = y?=w331:bool)
        n143 = Build Path(base path=w354, name or relative path=w355) -> (appended path=w334:path)
        n144 = call "Get Cluster Element Names.vi"("Cluster"=w352) -> ("Element Names"=w351:string[])  [unwired: 9 in, 1 out]
        n145 = Unbundle By Name(w352) -> ("Turb Stats"=w342:T4)
        n146 = call <vilib>:"Check if File or Folder Exists.vi"("path"=w334) -> ("file or folder exists?"=w332:bool, "dup path"=w333:path)  [unwired: 8 in, 1 out]
        n147 = And(x=w331, y=w332) -> (x .and. y?=w328:bool)
        n148 = case shown="True" w328 {
          tunnel: [w363 path "" ("dup path")] -> w320
          tunnel: w333 -> [w363 _]
          frame False {
          }
          frame True {
            w366 = T5 1 items=["no dialog", "OK message", "continue or stop message", "OK message + warnings", "continue/stop + warnings"] ("type of dialog (OK msg:1)")
            n149 = call <vilib>:"Simple Error Handler.vi"("type of dialog (OK msg:1)"=w366, "error in (no error)"=errorcluster {"status"=TRUE, "code"=0, "source"="Folder already exists, please select a new case name or results folder"}) -> ()  [unwired: 3 in, 5 out]
          }
        }
        n150 = Delete From Array(array=w351, length=10, index=1) -> (deleted portion=w339:string[], array with subset deleted=w347:string[])
        n151 = Index Array(array=w342) -> (element=w341:T3)  [unwired: 1 in]
        n152 = call "Get Cluster Element Names.vi"("Cluster"=w341) -> ("Element Names"=w348:string[])  [unwired: 9 in, 1 out]
        n153 = Delete From Array(array=w339, length=2, index=6) -> (deleted portion=w317:string[])  [unwired: 1 out]
        n154 = for {
          tunnel: w317 -> [w369] mode=indexing
          tunnel: w348 -> [w368]
          tunnel: [w367] -> w346 mode=indexing
          n155 = for {
            tunnel: w369 -> [w373]
            tunnel: w368 -> [w371] mode=indexing
            tunnel: [w370] -> w367 mode=indexing
            n156 = Concatenate Strings(w373, "_" ("string"), w371) -> (w370:string)
          }
        }
        n157 = Index Array(array=w346) -> (element #1=w345:string[], element #2=w344:string[])  [unwired: 4 in]
        n158 = Build Array (concatenate)(w347, w345, w344) -> (w343:string[])
        n159 = for {
          tunnel: w343 -> [w376] mode=indexing
          tunnel: [w378] -> w321 mode=indexing
          w382 = "_" ("Replace with")
          n160 = call <vilib>:"Trim Whitespace.vi"("string"=w376) -> ("trimmed string"=w374:string)  [unwired: 1 in]
          n161 = call "Replace_Character.vi"("Replace with"="_", "Input String"=w374, "Search For"=" ") -> ("Output string"=w377:string)  [unwired: 1 out]
          n162 = call "Replace_Character.vi"("Replace with"=w382, "Input String"=w377, "Search For"="(") -> ("Output string"=w384:string)  [unwired: 1 out]
          n163 = call "Replace_Character.vi"("Replace with"=w382, "Input String"=w384, "Search For"=")") -> ("Output string"=w381:string)  [unwired: 1 out]
          n164 = call "Replace_Character.vi"("Replace with"="", "Input String"=w381, "Search For"="/") -> ("Output string"=w378:string)  [unwired: 1 out]
        }
        "Variable Names" <- w321
        n165 = for {
          tunnel: w320 -> [w362]
          tunnel: [w356] -> w326 mode=indexing
          tunnel: w321 -> [_] mode=indexing
          i -> [w361]
          n166 = Increment(x=w361) -> (x+1=w360:i32)
          n167 = Number To Decimal String(number=w360) -> (decimal integer string=w358:string)  [unwired: 1 in]
          n168 = Concatenate Strings("ENSI.var" ("name or relative path"), w358) -> (w357:string)
          n169 = Build Path(base path=w362, name or relative path=w357) -> (appended path=w356:path)
        }
        n170 = Build Path(base path=w320, name or relative path="ENSI.case") -> (appended path=w324:path)
        n171 = Build Path(base path=w320, name or relative path="ENSI.geo") -> (appended path=w325:path)
        n172 = Build Array (concatenate)(w324, w325, w326) -> (→"File Paths":path[])
        n173 = Select(t="End Time", s=w328, f="Setup Files" ("t")) -> (s? t:f=w330:string)
      }
      frame "Setup Files" {
        n174 = local read "File Paths"() -> (w392:path[])
        n175 = local write "Status"("Setting up case files ready to write to..." ("Status")) -> ()
        n176 = for {
          N -> [w395]
          tunnel: w392 -> [w398] mode=indexing
          i -> [w393]
          n177 = Divide(x=w393, y=w395) -> (x/y=w394:dbl)
          n178 = Multiply(x=w394, y=100) -> (x*y=w397:dbl)
          n179 = local write "Progress Bar"(w397) -> ()
          n180 = case shown="0" w393 {
            tunnel: w398 -> [w403 w424 w443]
            tunnel: w393 -> [_ _ w438]
            frame 0 {
              n181 = local read "Variable Names"() -> (w400:string[])
              n182 = for {
                tunnel: w400 -> [w409] mode=indexing
                tunnel: [w407] -> w399 mode=indexing
                i -> [w412]
                n183 = Increment(x=w412) -> (x+1=w413:i32)
                n184 = Number To Decimal String(number=w413) -> (decimal integer string=w410:string)  [unwired: 1 in]
                n185 = Concatenate Strings(" ENSI.var", w410) -> (w408:string)
                n186 = Concatenate Strings("scalar per node: ", w409, w408) -> (w407:string)
              }
              n187 = Build Array (concatenate)(string[] ["FORMAT", "type: ensight gold", "GEOMETRY", "model: ENSI.geo", "VARIABLE"], w399) -> (w402:string[])
              n188 = for {
                tunnel: w402 -> [w419] mode=indexing
                shift-right: [w417] -> w405
                shift-left: "" -> [w415]
                n189 = Concatenate Strings(w419, "\r\n") -> (w416:string)
                n190 = Concatenate Strings(w415, w416) -> (w417:string)
              }
              n191 = call "Write_File_Simple.vi"("append to file? (new file:F)"=FALSE, "character string"=w405, "file path"=w403) -> ()  [unwired: 2 out]
            }
            frame 1 {
              n192 = local read "# total vectors"() -> (w422:i32)
              n193 = Number To Decimal String(number=w422) -> (decimal integer string=w421:string)  [unwired: 1 in]
              n194 = Build Array (concatenate)(string[] ["EnSight Model Geometry File", "EnSight 9.2 ", "node id assign", "element id assign", "part", "         1", "Point field", "coordinates"], w421) -> (w420:string[])
              n195 = for {
                tunnel: w420 -> [w432] mode=indexing
                shift-right: [w430] -> w426
                shift-left: "" -> [w428]
                n196 = Concatenate Strings(w432, "\r\n") -> (w429:string)
                n197 = Concatenate Strings(w428, w429) -> (w430:string)
              }
              n198 = call "Write_File_Simple.vi"("append to file? (new file:F)"=FALSE, "character string"=w426, "file path"=w424) -> ()  [unwired: 2 out]
            }
            frame 2, Default {
              n199 = local read "Variable Names"() -> (w439:string[])
              n200 = Subtract(x=w438, y=2) -> (x-y=w436:i32)
              n201 = Index Array(array=w439, index=w436) -> (element=w435:string)
              n202 = Build Array (concatenate)(w435, string[] ["part", "         1", "coordinates"]) -> (w433:string[])
              n203 = for {
                tunnel: w433 -> [w448] mode=indexing
                shift-right: [w446] -> w441
                shift-left: "" -> [w444]
                n204 = Concatenate Strings(w448, "\r\n") -> (w445:string)
                n205 = Concatenate Strings(w444, w445) -> (w446:string)
              }
              n206 = call "Write_File_Simple.vi"("append to file? (new file:F)"=FALSE, "character string"=w441, "file path"=w443) -> ()  [unwired: 2 out]
            }
          }
        }
      }
      frame "Collect Data" {
        w453 = T2 []  # Array
        n207 = for {
          N -> [w467]
          tunnel: w455 -> [w475] mode=indexing
          tunnel: [w473] -> w449 mode=indexing
          tunnel: [w472] -> w451 mode=indexing
          i -> [w468]
          w459 = 1 ("n")
          n208 = Unbundle By Name(w475) -> ("Record Length"=w474:dbl, "Turb Stats"=w458:T4, "Turb Stats Error"=w461:T4, "XYZ Position"=w472:dbl[])
          n209 = Divide(x=w468, y=w467) -> (x/y=w470:dbl)
          n210 = Multiply(x=w470, y=100) -> (x*y=w471:dbl)
          n211 = local write "Progress Bar"(w471) -> ()
          n212 = Rotate 1D Array(1:w461, 2:w459) -> (0:w462:T4)
          n213 = Rotate 1D Array(1:w458, 2:w459) -> (0:w460:T4)
          n214 = Index Array(array=w460) -> (element=w466:T3)  [unwired: 1 in]
          n215 = Index Array(array=w462) -> (element=w464:T3)  [unwired: 1 in]
          n216 = Cluster To Array(cluster=w466) -> (array=w465:dbl[])
          n217 = Cluster To Array(cluster=w464) -> (array=w463:dbl[])
          n218 = Build Array (concatenate)(w474, w465, w463) -> (w473:dbl[])
        }
        "Data Array (spot,Var)" <- w449
        n219 = local write "Status"("Gathering all the data ready to write to file..." ("Status")) -> ()
        n220 = Transpose 2D Array(2D array=w451) -> (transposed array=→"Position Array (XYZ,spot)":dbl[][])
      }
      frame "Save Data" {
        n221 = local read "Data Array (spot,Var)"() -> (w480:dbl[][])
        n222 = local read "Position Array (XYZ,spot)"() -> (w479:dbl[][])
        n223 = local read "File Paths"() -> (w481:path[])
        n224 = Transpose 2D Array(2D array=w480) -> (transposed array=w476:dbl[][])
        n225 = local write "Status"("Wrting the data to file..." ("Status")) -> ()
        n226 = for {
          N -> [w485]
          tunnel: w481 -> [w492] mode=indexing
          tunnel: w476 -> [w491]
          tunnel: w479 -> [w490]
          i -> [w486]
          # "Loop Variable"
          n227 = Divide(x=w486, y=w485) -> (x/y=w488:dbl)
          n228 = Multiply(x=w488, y=100) -> (x*y=w489:dbl)
          n229 = local write "Progress Bar"(w489) -> ()
          n230 = case shown="2, Default" w486 {
            tunnel: w492 -> [_ w498 w510]
            tunnel: w486 -> [_ _ w517]
            tunnel: w491 -> [_ _ w514]
            tunnel: w490 -> [_ w497 _]
            frame 0 {
            }
            frame 1 {
              n231 = Index Array(array=w497) -> (element #1=w496:dbl[], element #2=w495:dbl[], element #3=w494:dbl[])  [unwired: 6 in]
              n232 = Build Array (concatenate)(w496, w495, w494) -> (w493:dbl[])
              n233 = for {
                tunnel: w493 -> [w502] mode=indexing
                shift-right: [w508] -> w499
                shift-left: "" -> [w507]
                w503 = T5 4 items=["no dialog", "OK message", "continue or stop message", "OK message + warnings", "continue/stop + warnings"] ("type of dialog (OK msg:1)")
                n234 = call "Ensight_Format_Check.vi"("Input Number"=w502) -> ("error"=w505:errorcluster, "Output string"=w506:string)  [unwired: 8 in, 1 out]
                n235 = Concatenate Strings(w507, w506) -> (w508:string)
                n236 = call <vilib>:"Simple Error Handler.vi"("error source (\" \")"="GEOM" ("error source (\" \")"), "type of dialog (OK msg:1)"=w503, "error in (no error)"=w505) -> ()  [unwired: 2 in, 5 out]
              }
              n237 = call "Write_File_Simple.vi"("append to file? (new file:F)"=TRUE, "character string"=w499, "file path"=w498) -> ()  [unwired: 2 out]
            }
            frame 2, Default {
              n238 = Subtract(x=w517, y=2) -> (x-y=w509:i32)
              n239 = Index Array(array=w514, index (row)=w509) -> (element=w513:dbl[])  [unwired: 1 in]
              n240 = for {
                tunnel: w513 -> [w518] mode=indexing
                shift-right: [w527] -> w511
                shift-left: "" -> [w526]
                tunnel: w510 -> [w523]
                w519 = T5 4 items=["no dialog", "OK message", "continue or stop message", "OK message + warnings", "continue/stop + warnings"] ("type of dialog (OK msg:1)")
                n241 = Path To String(path=w523) -> (string=w522:string)
                n242 = call "Ensight_Format_Check.vi"("Input Number"=w518) -> ("error"=w524:errorcluster, "Output string"=w525:string)  [unwired: 8 in, 1 out]
                n243 = Concatenate Strings("VAR file: " ("error source (\" \")"), w522) -> (w520:string)
                n244 = call <vilib>:"Simple Error Handler.vi"("error source (\" \")"=w520, "type of dialog (OK msg:1)"=w519, "error in (no error)"=w524) -> ()  [unwired: 2 in, 5 out]
                n245 = Concatenate Strings(w526, w525) -> (w527:string)
              }
              n246 = call "Write_File_Simple.vi"("append to file? (new file:F)"=TRUE, "character string"=w511, "file path"=w510) -> ()  [unwired: 2 out]
            }
          }
        }
      }
      frame "End Time" {
        n247 = local write "Position Array (XYZ,spot)"(dbl[][] [] ("Position Array")) -> ()
        n248 = local write "Data Array (spot,Var)"(dbl[][] [] ("Data Array")) -> ()
      }
    }
  }
  "Progress Bar" <- u8 0 ("Progress Bar")
